vi "RT-Main_withPID.vi"() -> ()   [LabVIEW 2018]
uses:
  <vilib>/Studica/Studica Toolkit/Background/I2C Channel.ctl
  <vilib>/Studica/Studica Toolkit/Background/Mxp Selection.ctl
  <vilib>/robotics/Steering/Wheel/Rotation Direction.ctl
  <vilib>/robotics/Steering/Wheel/Wheel Parameters.ctl
  <vilib>/robotics/Steering/Omnidirectional Wheel/NI_Robotics_Omnidirectional Wheel.lvclass
  C:/Program Files (x86)/National Instruments/LabVIEW 2018/vi.lib/robotics/Steering/Wheel/NI_Robotics_Wheel.lvclass
  <vilib>/robotics/Steering/Omnidirectional Wheel/Create Omnidirectional Wheel.vi
  <vilib>/robotics/Steering/Steering Frame/Create User Defined Steering Frame.vi
  <vilib>/robotics/Steering/Steering Frame/Apply Steering Frame Velocity to Motors.vi
  <vilib>/robotics/Steering/Steering Frame/NI_Robotics_Steering Frame.lvclass
  <vilib>/robotics/Steering/Wheel/NI_Robotics_Wheel.lvclass
  <vilib>/Studica/Studica Toolkit/NavX/NavX.lvlib
  <vilib>/Studica/Studica Blackhawk/Blackhawk.lvlib
panel:
  in  "Robot Facing":i16=4
  out "data out":T1(array[cluster])
  in  "NavX PID gains":T2(array[cluster])=[{"proportional gain (Kc)"=0.15, "integral time (Ti, min)"=0.0, "derivative time (Td, min)"=0.003}] {"integral time (Ti, min)" min=0.0 step=0.0001}
  out "Angular velocity setpoint":dbl
  out "YRPHfH":T3={"Yaw"=0.15, "Roll"=2.38, "Pitch"=-4.28, "Heading"=48.3, "Fused Heading"=0.15}
  out "error out":errorcluster
  in  "Angular Velocity (rad/s)":dbl(slide)=-0.0 min=-1.0 max=1.0 scale=1.0..-1.0
  in  "Y Velocity (m/s)":dbl(slide)=-0.0 min=-1.0 max=1.0 scale=-1.0..1.0
  in  "X Velocity (m/s)":dbl(slide)=-0.0 min=-1.0 max=1.0 scale=-1.0..1.0
  in  "Wheel Index Adjustment":i32[](array[numeric])=[2, 0, 1]
  out "Desired Velocity":dbl[](array[numeric])=[0.0033749999999999995, 0.0033749999999999995, 0.0033749999999999995]
  out "PID-Output":dbl[](array[numeric])=[0.004570312508683128, 0.004570312508683128, 0.004570312508683128, 0.004570312508683128]
  in  "PID gains":T2(array[cluster])=[{"proportional gain (Kc)"=1.3, "integral time (Ti, min)"=0.004, "derivative time (Td, min)"=0.0}, {"proportional gain (Kc)"=1.3, "integral time (Ti, min)"=0.004, "derivative time (Td, min)"=0.0}, {"proportional gain (Kc)"=1.3, "integral time (Ti, min)"=0.004, "derivative time (Td, min)"=0.0}] {"proportional gain (Kc)" step=0.01; "integral time (Ti, min)" min=0.0 step=0.0001; "derivative time (Td, min)" step=0.0001}
  in  "Reset Encoders":bool
  out "Actual-SpeedList":dbl[](array[numeric])
  out "Tick Count(uSec)":u32=10160615 caption="Tick Count(Ticks)"
  in  "Speed M1":dbl(slide) scale=-1.0..1.0
  in  "StopMotors":bool
  in  "Stop Program":bool
  in  "Robot Model":string(combo)="3-wheeled"
  out "timed out?":bool
  out "available IP addresses":string[](array[string])=["172.16.0.1", "127.0.0.1"]
  # "Configuration"
  # "Speed related shit"
  # "Controller"
  # "NAVX data"
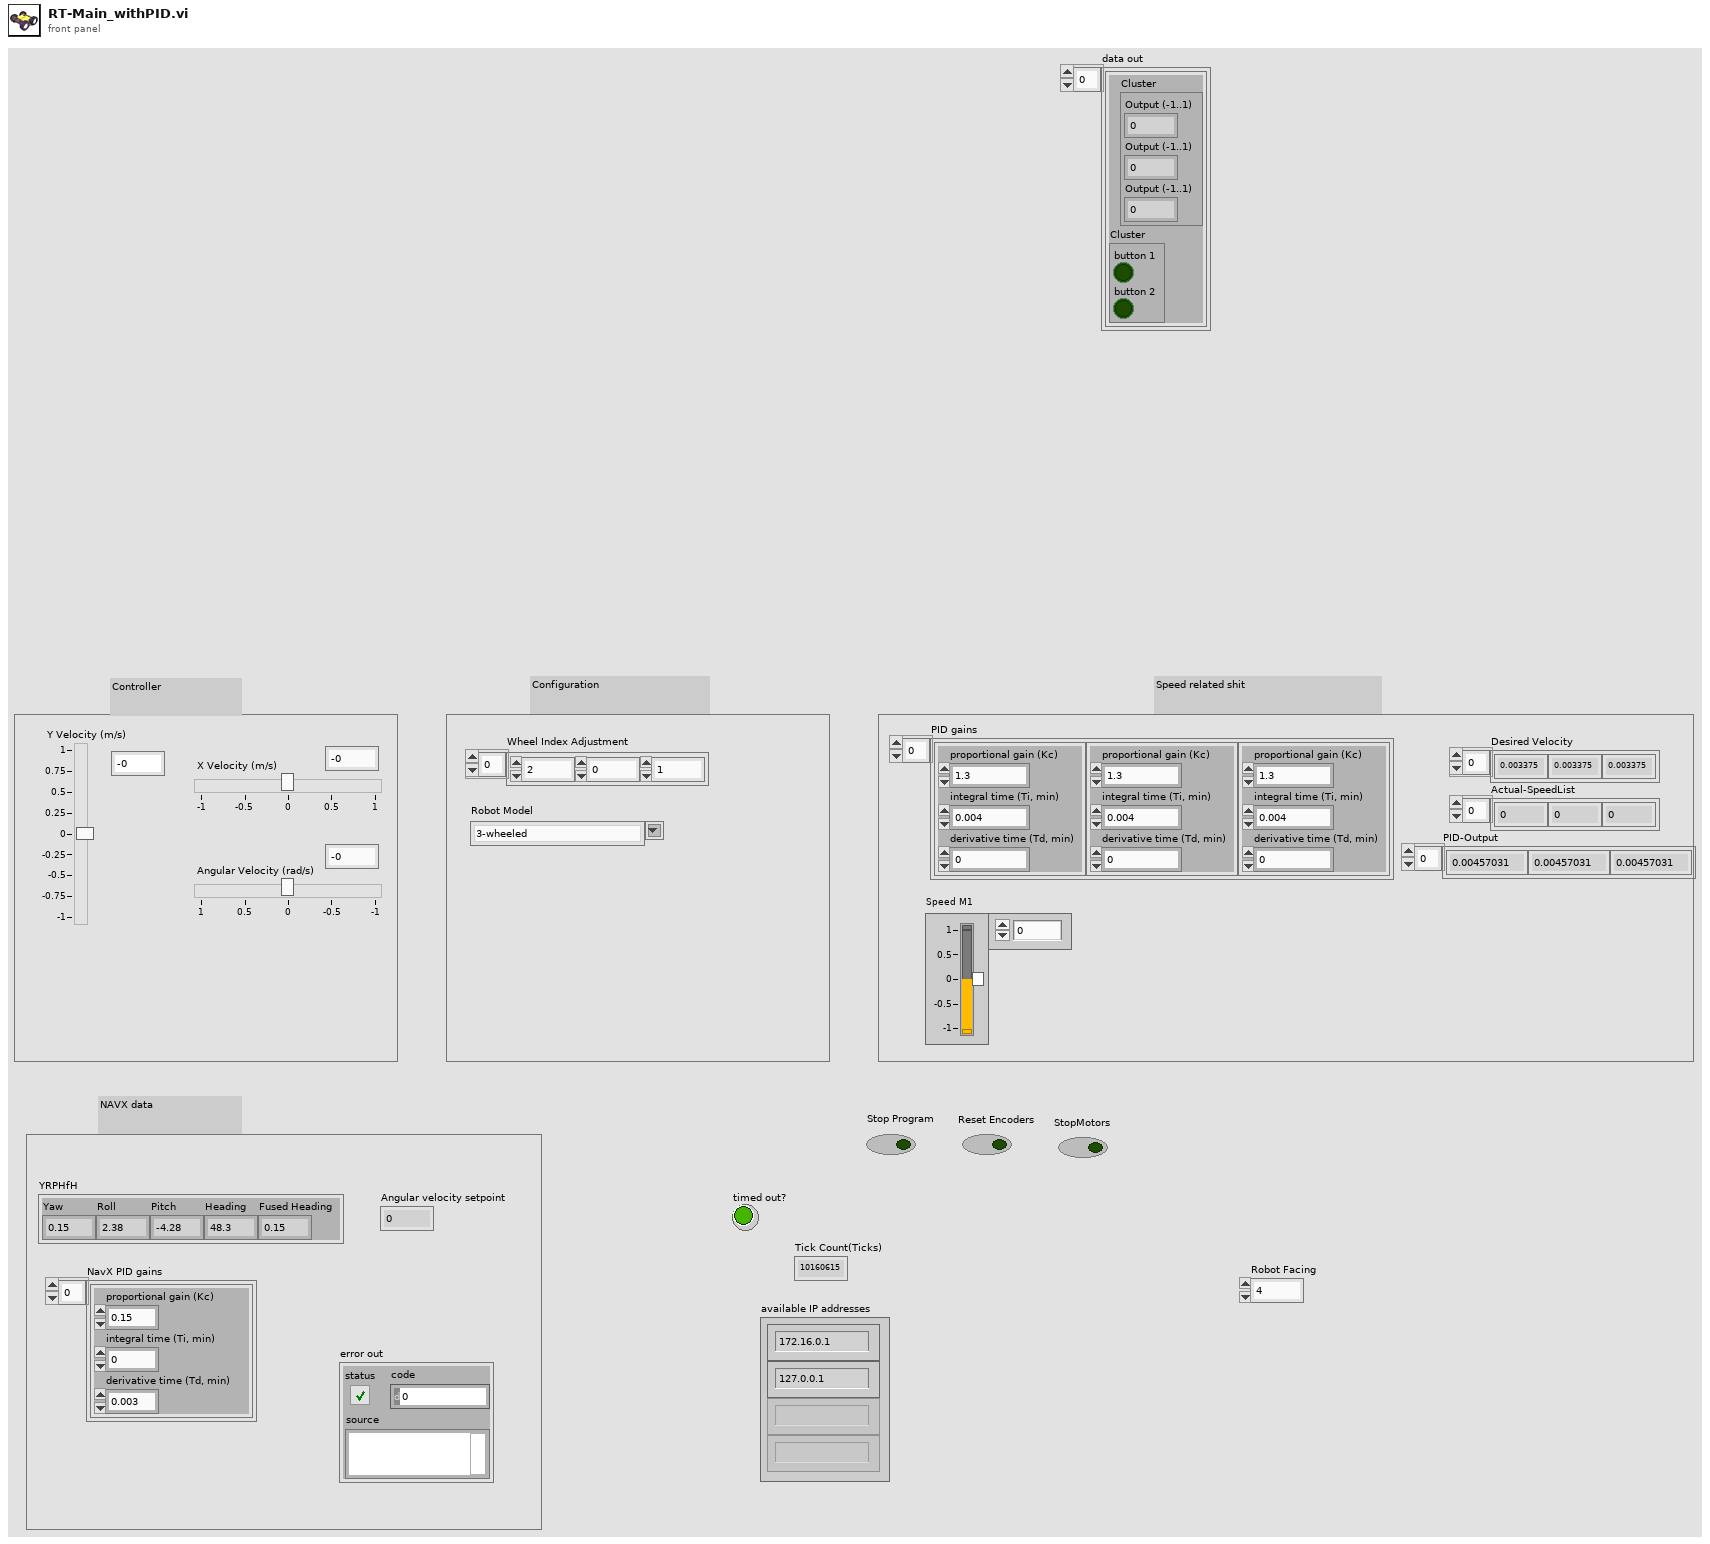
[diagram p1: front panel]
types:
  T1 = cluster{"Cluster":cluster{"Output (-1..1)":dbl, "Output (-1..1)":dbl, "Output (-1..1)":dbl}, "Cluster":cluster{"button 1":bool, "button 2":bool}}[]
  T2 = cluster{"proportional gain (Kc)":dbl, "integral time (Ti, min)":dbl, "derivative time (Td, min)":dbl}[]
  T3 = cluster{"Yaw":dbl, "Roll":dbl, "Pitch":dbl, "Heading":dbl, "Fused Heading":dbl}
  T4 = typedef "I2C Channel.ctl" = enum16{"Not Connected", "A", "B"}
  T5 = cluster{"Cluster":cluster{"Output (-1..1)":dbl, "Output (-1..1)":dbl, "Output (-1..1)":dbl}, "Cluster":cluster{"button 1":bool, "button 2":bool}}
  T6 = cluster{"Output (-1..1)":dbl, "Output (-1..1)":dbl, "Output (-1..1)":dbl}
  T7 = typedef "Mxp Selection.ctl" = enum16{"MXP A", "MXP B"}
  T8 = typedef "I2C.lvlib/I2C Reference.ctl" = cluster{"myRIO Reference":T9, "I2C Channels Enum":T13, "I2C Configuration":T14}
  T9 = typedef "myRIO Generic Hardware Reference.ctl" = cluster{"myRIO Model":T10, "myRIO Hardware Reference":T11}
  T10 = typedef "Hardware Version Enum.ctl" = enum16{"Unknown", "myRIO-1900", "myRIO-1950", "roboRIO", "NI ELVIS RIO CM", "ELVIS III"}
  T11 = typedef "myRIO v1.0 Reference.ctl" = cluster{"Generic FPGA Reference":T12, "Allow multiple opens":bool}
  T12 = typedef "Generic FPGA Reference.ctl" = refnum<k20>
  T13 = typedef "I2C Channels Enum.ctl" = enum16{"Not Connected", "A/I2C", "B/I2C", "I2C/I2C"}
  T14 = typedef "I2C.lvlib/I2C Configuration.ctl" = cluster{"I2C Transfer Rate":T15}
  T15 = typedef "I2C.lvlib/I2C Transfer Rate.ctl" = enum16{"Standard mode (100 kbps)", "Fast mode (400 kbps)"}
  T16 = cluster{"I2C Ref Out":cluster{"I2C Channel":T4, "FPGA VI Reference Out":refnum<k20>}, "Connected":bool, "Slave Address (7-bit)":u8, "Registry":u8[]}
  T17 = typedef "NI_Robotics_Wheel.lvclass/Wheel Parameters.ctl" = cluster{"wheel radius":dbl, "gear ratio":dbl, "forward rotation direction":T18}
  T18 = typedef "NI_Robotics_Wheel.lvclass/Rotation Direction.ctl" = u16
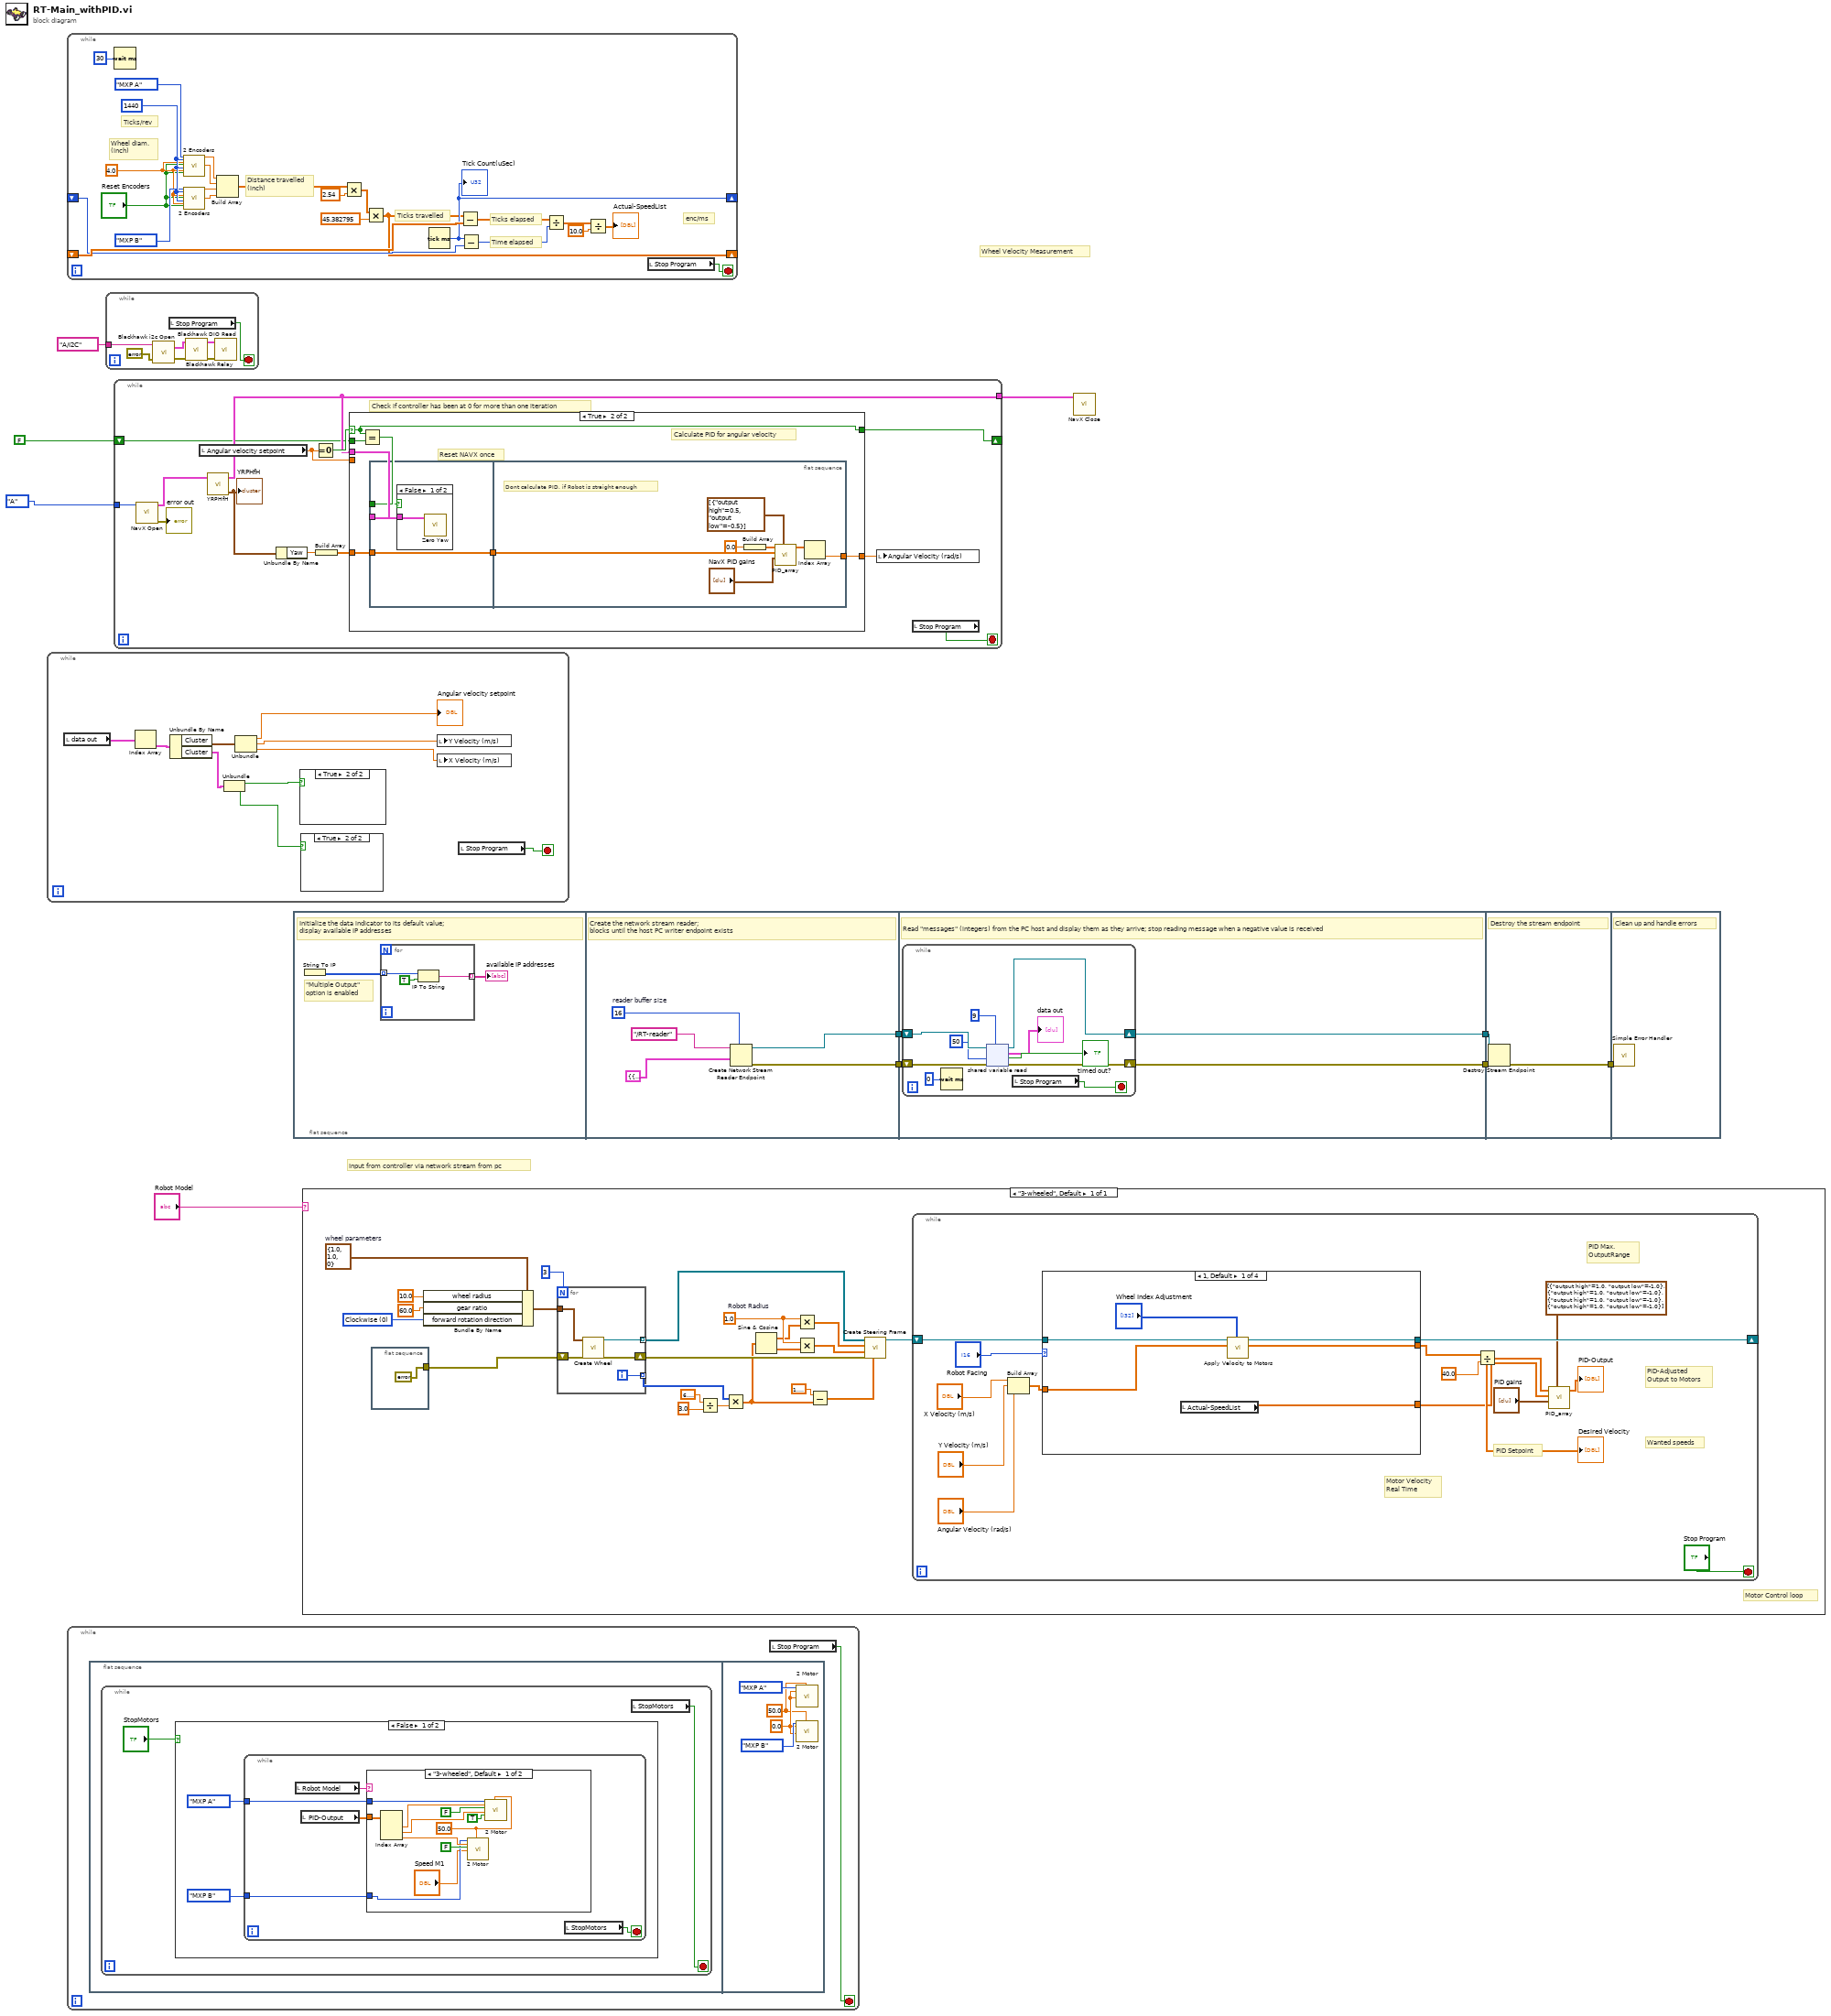
[diagram p0: block diagram]
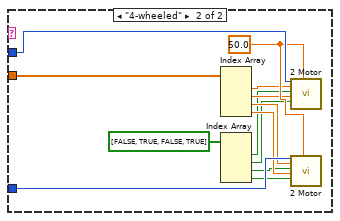
[diagram p6: hidden frame]
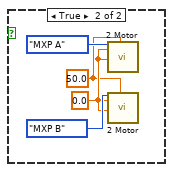
[diagram p7: hidden frame]
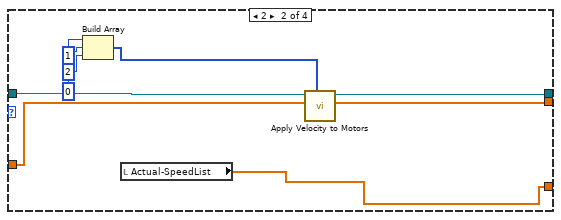
[diagram p8: hidden frame]
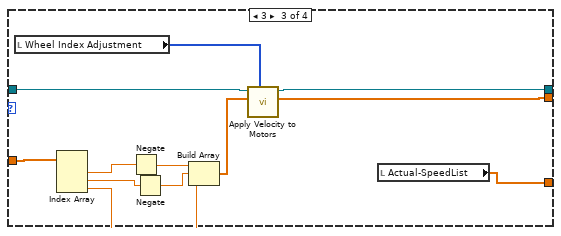
[diagram p9: hidden frame]
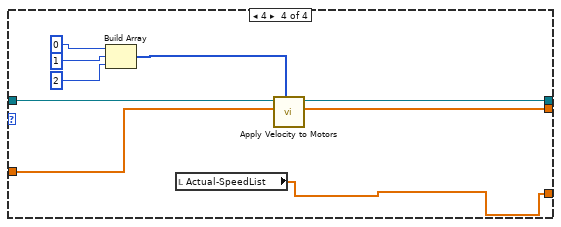
[diagram p10: hidden frame]
diagram:
  # "Input from controller via network stream from pc"
  # "Wheel Velocity Measurement"
  n1 = while {
    stop <- w20 stop-if-true
    n2 = local read "data out"() -> (w19:T1)
    n3 = Index Array(array=w19) -> (element=w18:T5)  [unwired: 1 in]
    n4 = Unbundle By Name(w18) -> ("Cluster"=w17:T6, "Cluster"=w13:cluster{"button 1":bool, "button 2":bool})
    n5 = Unbundle(w13) -> ("button 1"=w12:bool, "button 2"=w11:bool)
    n6 = Unbundle(w17) -> ("Output (-1..1)"=→"Angular velocity setpoint":dbl, "Output (-1..1)"=w15:dbl, "Output (-1..1)"=w14:dbl)
    n7 = case shown="True" w12 {
      frame False {
      }
      frame True {
      }
    }
    n8 = case shown="True" w11 {
      frame False {
      }
      frame True {
      }
    }
    n9 = local write "Y Velocity (m/s)"(w15) -> ()
    n10 = local write "X Velocity (m/s)"(w14) -> ()
    n11 = local read "Stop Program"() -> (w20:bool)
  }
  n12 = while {
    shift-right: [w28] -> _
    shift-left: _ -> [w33]
    shift-right: [w29] -> _
    shift-left: _ -> [w31]
    stop <- w21 stop-if-true
    w26 = 4.0 ("Wheel Diameter M1 (inches)")
    w36 = u32 1440 ("Ticks Per Rev M0")
    # "Ticks travelled"
    # "Distance travelled\n(inch)"
    # "Wheel diam.\n(inch)"
    # "Ticks/rev"
    # "Ticks elapsed"
    # "Time elapsed"
    # "enc/ms"
    n13 = Wait (ms)(milliseconds to wait=u32 30) -> ()  [unwired: 1 out]
    n14 = call <vilib>:"2 Encoders.vi"("Mxp Side"=Mxp_Selection."MXP A", "Ticks Per Rev M0"=w36, "Wheel Diameter M0 (inches)"=w26, "Reset Encoder 0"="Reset Encoders", "Ticks Per Rev M1"=w36, "Wheel Diameter M1 (inches)"=w26, "Reset Encoder 1"="Reset Encoders") -> ("Distance M0 (inches)"=w37:dbl, "Distance M1 (inches)"=w38:dbl)  [unwired: 18 in, 1 out]
    n15 = call <vilib>:"2 Encoders.vi"("Mxp Side"=Mxp_Selection."MXP B", "Ticks Per Rev M0"=w36, "Wheel Diameter M0 (inches)"=w26, "Reset Encoder 0"="Reset Encoders", "Ticks Per Rev M1"=w36, "Wheel Diameter M1 (inches)"=w26, "Reset Encoder 1"="Reset Encoders") -> ("Distance M0 (inches)"=w39:dbl, "Distance M1 (inches)"=w27:dbl)  [unwired: 18 in, 1 out]
    n16 = Build Array(w37, w38, w39, w27) -> (w41:dbl[])
    n17 = Multiply(x=w41, y=2.54) -> (x*y=w42:dbl[])
    n18 = Multiply(x=w42, y=45.382795) -> (x*y=w28:dbl[])
    n19 = Tick Count (ms)() -> (millisecond timer value=w29:u32)
    "Tick Count(uSec)" <- w29
    n20 = Subtract(x=w28, y=w33) -> (x-y=w32:dbl[])
    n21 = Subtract(x=w29, y=w31) -> (x-y=w44:u32)
    n22 = Divide(x=w32, y=w44) -> (x/y=w24:dbl[])
    n23 = Divide(x=w24, y=10.0) -> (x/y=→"Actual-SpeedList":dbl[])
    n24 = local read "Stop Program"() -> (w21:bool)
  }
  n25 = while {
    stop <- w45 stop-if-true
    n26 = flat-sequence {
      frame #0 {
        n27 = while {
          stop <- w46 stop-if-true
          n28 = case shown="False" "StopMotors" {
            frame False {
              n29 = while {
                tunnel: Mxp_Selection."MXP A" ("Mxp Side") -> [w54]
                tunnel: Mxp_Selection."MXP B" ("Mxp Side") -> [w53]
                stop <- w50 stop-if-true
                n30 = local read "Robot Model"() -> (w52:string)
                n31 = local read "PID-Output"() -> (w51:dbl[])
                n32 = case shown="\"3-wheeled\", Default" w52 {
                  tunnel: w54 -> [w57 w78]
                  tunnel: w53 -> [w56 w77]
                  tunnel: w51 -> [w58 w66]
                  frame "3-wheeled", Default {
                    w65 = 50.0 ("Frequency [Hz]")
                    n33 = Index Array(array=w58) -> (element #1=w61:dbl, element #2=w60:dbl, element #3=w59:dbl)  [unwired: 3 in]
                    n34 = call <vilib>:"2 Motor.vi"("Mxp Side"=w56, "Speed M0"=w59, "Invert M0"=FALSE, "Speed M1"="Speed M1", "Frequency [Hz]"=w65) -> ()  [unwired: 14 in, 1 out]
                    n35 = call <vilib>:"2 Motor.vi"("Mxp Side"=w57, "Speed M0"=w61, "Invert M0"=FALSE, "Speed M1"=w60, "Invert M1"=TRUE ("Invert M0"), "Frequency [Hz]"=w65) -> ()  [unwired: 13 in, 1 out]
                  }
                  frame "4-wheeled" {
                    w76 = 50.0 ("Frequency [Hz]")
                    n36 = Index Array(array=w66) -> (element #1=w75:dbl, element #2=w74:dbl, element #3=w73:dbl, element #4=w72:dbl)  [unwired: 4 in]
                    n37 = Index Array(array=bool[] [FALSE, TRUE, FALSE, TRUE] ("Motor Directions")) -> (element #1=w70:bool, element #2=w69:bool, element #3=w68:bool, element #4=w67:bool)  [unwired: 4 in]
                    n38 = call <vilib>:"2 Motor.vi"("Mxp Side"=w78, "Speed M0"=w75, "Invert M0"=w70, "Speed M1"=w74, "Invert M1"=w69, "Frequency [Hz]"=w76) -> ()  [unwired: 13 in, 1 out]
                    n39 = call <vilib>:"2 Motor.vi"("Mxp Side"=w77, "Speed M0"=w73, "Invert M0"=w68, "Speed M1"=w72, "Invert M1"=w67, "Frequency [Hz]"=w76) -> ()  [unwired: 13 in, 1 out]
                  }
                }
                n40 = local read "StopMotors"() -> (w50:bool)
              }
            }
            frame True {
              w79 = 50.0 ("Frequency [Hz]")
              w80 = 0.0 ("Speed M0")
              n41 = call <vilib>:"2 Motor.vi"("Mxp Side"=Mxp_Selection."MXP A", "Speed M0"=w80, "Speed M1"=w80, "Frequency [Hz]"=w79) -> ()  [unwired: 15 in, 1 out]
              n42 = call <vilib>:"2 Motor.vi"("Mxp Side"=Mxp_Selection."MXP B", "Speed M0"=w80, "Speed M1"=w80, "Frequency [Hz]"=w79) -> ()  [unwired: 15 in, 1 out]
            }
          }
          n43 = local read "StopMotors"() -> (w46:bool)
        }
      }
      frame #1 {
        w83 = 50.0 ("Frequency [Hz]")
        w84 = 0.0 ("Speed M0")
        n44 = call <vilib>:"2 Motor.vi"("Mxp Side"=Mxp_Selection."MXP A", "Speed M0"=w84, "Speed M1"=w84, "Frequency [Hz]"=w83) -> ()  [unwired: 15 in, 1 out]
        n45 = call <vilib>:"2 Motor.vi"("Mxp Side"=Mxp_Selection."MXP B", "Speed M0"=w84, "Speed M1"=w84, "Frequency [Hz]"=w83) -> ()  [unwired: 15 in, 1 out]
      }
    }
    n46 = local read "Stop Program"() -> (w45:bool)
  }
  n47 = while {
    tunnel: tag "A/I2C" ("Channel Name") -> [w93]
    stop <- w92 stop-if-true
    n48 = call <vilib>:"Blackhawk i2c Open.vi"("error in (no error)"=errorcluster {"status"=FALSE, "code"=0, "source"=""}, "Channel Name"=w93) -> ("error out"=w89:errorcluster, "I2C Ref Out"=w90:T8)  [unwired: 2 in]
    n49 = local read "Stop Program"() -> (w92:bool)
    n50 = call <vilib>:"Blackhawk Relay.vi"("error in (no error)"=w89, "I2C Ref In"=w90) -> ("error out"=w87:errorcluster, "I2C Ref Out"=w88:T8)  [unwired: 8 in]
    n51 = call <vilib>:"Blackhawk DIO Read.vi"("I2C Ref In"=w88, "error in (no error)"=w87) -> ()  [unwired: 4 in, 3 out]
  }
  n52 = while {
    tunnel: [w98] -> w4
    shift-right: [w96] -> _
    shift-left: FALSE -> [w95]
    tunnel: I2C_Channel."A" ("I2C Channel") -> [w94]
    stop <- w106 stop-if-true
    # "Check if controller has been at 0 for more than one iteration"
    n53 = call <vilib>:"NavX Open.vi"("I2C Channel"=w94) -> ("error out"=→"error out":errorcluster, "NavX Info"=w104:T16)  [unwired: 9 in]
    n54 = local read "Angular velocity setpoint"() -> (w97:dbl)
    n55 = call <vilib>:"YRPHfH.vi"("NavX Info In"=w104) -> ("YRPHfH"=w103:T3, "NavX Info Out"=w98:T16)  [unwired: 3 in]
    "YRPHfH" <- w103
    n56 = Unbundle By Name(w103) -> ("Yaw"=w99:dbl)
    n57 = Equal To 0?(x=w97) -> (x = 0?=w100:bool)
    n58 = Build Array(w99) -> (w102:dbl[])
    n59 = case shown="True" w100 {
      selector: w100 -> [w107 w111]
      tunnel: w102 -> [_ w114]
      tunnel: [w108 w115] -> w101
      tunnel: w98 -> [_ w112]
      tunnel: w97 -> [w108 _]
      tunnel: [w107 w111] -> w96
      tunnel: w95 -> [_ w110]
      frame False {
        # "Adjust angular velocity if controller != 0"
      }
      frame True {
        # "Reset NAVX once"
        # "Calculate PID for angular velocity"
        n60 = Equal?(x=w111, y=w110) -> (x = y?=w109:bool)
        n61 = flat-sequence {
          tunnel: [w118] -> w113
          tunnel: w114 -> [w118]
          tunnel: w112 -> [w117]
          tunnel: w109 -> [w116]
          tunnel: [w126] -> w115
          tunnel: w113 -> [w125]
          frame #0 {
            n62 = case shown="False" w116 {
              tunnel: w117 -> [w119 _]
              frame False {
                n63 = call <vilib>:"Zero Yaw.vi"("NavX Info In"=w119) -> ()  [unwired: 10 in, 1 out]
              }
              frame True {
              }
            }
          }
          frame #1 {
            # "Dont calculate PID, if Robot is straight enough"
            n64 = Build Array(0.0 ("element")) -> (w123:dbl[])
            n65 = call "PID_array.vi"("output range"=cluster{"output high":dbl, "output low":dbl}[] [{"output high"=0.5, "output low"=-0.5}], "PID gains"="NavX PID gains", "process variable"=w125, "setpoint"=w123) -> ("output"=w124:dbl[])  [unwired: 6 in, 1 out]
            n66 = Index Array(array=w124) -> (element=w126:dbl)  [unwired: 1 in]
          }
        }
      }
    }
    n67 = local write "Angular Velocity (rad/s)"(w101) -> ()
    n68 = local read "Stop Program"() -> (w106:bool)
  }
  n69 = flat-sequence {
    tunnel: [w134] -> w10
    tunnel: [w133] -> w9
    tunnel: [w137] -> w8
    tunnel: [w138] -> w7
    tunnel: w10 -> [w139]
    tunnel: w9 -> [w140]
    tunnel: w8 -> [w153]
    tunnel: w7 -> [w152]
    tunnel: [w151] -> w6
    tunnel: w6 -> [w154]
    frame #0 {
      # "\"Multiple Output\"\noption is enabled"
      # "Initialize the data indicator to its default value;\ndisplay available IP addresses"
      n70 = String To IP() -> (0:w127:u32[])  [unwired: 1 in]
      n71 = for {
        tunnel: w127 -> [w130] mode=indexing
        tunnel: [w129] -> w128 mode=indexing
        n72 = IP To String(1:TRUE ("dot notation? (F)"), 2:w130) -> (0:w129:string)
      }
      "available IP addresses" <- w128
    }
    frame #1 {
      w136 = 16  # reader buffer size
      # "Create the network stream reader;\nblocks until the host PC writer endpoint exists"
      n73 = Create Network Stream Reader Endpoint(7:w136, 9:T5 {"Cluster"={"Output (-1..1)"=0.0, "Output (-1..1)"=0.0, "Output (-1..1)"=0.0}, "Cluster"={"button 1"=FALSE, "button 2"=FALSE}} ("Controller Values"), 11:"/RT-reader" ("writer name")) -> (0:w134:errorcluster, 3:w133:refnum<k21>)  [unwired: 4 in]
    }
    frame #2 {
      # "Read \"messages\" (integers) from the PC host and display them as they arrive; stop reading message when a negative value is received"
      n74 = while {
        shift-right: [w148] -> w137
        shift-left: w140 -> [w150]
        shift-right: [w144] -> w138
        shift-left: w139 -> [w147]
        stop <- w142 stop-if-true
        n75 = Wait (ms)(milliseconds to wait=u32 0) -> ()  [unwired: 1 out]
        n76 = shared-variable-read(w150, w147, 50 ("timeout ms (-1)"), 9 ("# elements")) -> (w148:refnum<k21>, w144:errorcluster, →"timed out?":bool, →"data out":T1)
        n77 = local read "Stop Program"() -> (w142:bool)
      }
    }
    frame #3 {
      # "Destroy the stream endpoint"
      n78 = Destroy Stream Endpoint(8:w152, 11:w153) -> (0:w151:errorcluster)
    }
    frame #4 {
      # "Clean up and handle errors"
      n79 = call <vilib>:"Simple Error Handler.vi"("error in (no error)"=w154) -> ()  [unwired: 4 in, 5 out]
    }
  }
  n80 = case shown="\"3-wheeled\", Default" "Robot Model" {
    frame "3-wheeled", Default {
      w176 = T17 {"wheel radius"=1.0, "gear ratio"=1.0, "forward rotation direction"=0}  # wheel parameters
      w161 = T18 0 items=["Clockwise", "Counterclockwise"] ("forward rotation direction")
      w166 = 1.0  # Robot Radius
      # "Motor Control loop"
      n81 = flat-sequence {
        tunnel: [errorcluster {"status"=FALSE, "code"=0, "source"=""} ("error out")] -> w172
        frame #0 {
        }
      }
      n82 = Bundle By Name(cluster=w176, "wheel radius"=10.0, "gear ratio"=60.0, "forward rotation direction"=w161) -> (w173:T17)
      n83 = for {
        N: 3 -> [_]
        shift-right: [w232] -> w159
        shift-left: w172 -> [w233]
        tunnel: [w231] -> w171 mode=indexing
        tunnel: w173 -> [w230]
        tunnel: [w229] -> w167 mode=indexing
        i -> [w229]
        n84 = call-poly <vilib>:"Create Wheel.vi"("error in (no error)"=w233, "wheel parameters"=w230) -> ("error out"=w232:errorcluster, "omni wheel out"=w231:refnum<class "NI_Robotics_Omnidirectional Wheel.lvclass">)  [unwired: 8 in]
      }
      n85 = Divide(x=6.283185307179586, y=3.0) -> (x/y=w168:dbl)
      n86 = Multiply(x=w167, y=w168) -> (x*y=w156:dbl[])
      n87 = Sine & Cosine(0:w156) -> (1:w158:dbl[], 2:w157:dbl[])
      n88 = Multiply(x=w166, y=w158) -> (x*y=w165:dbl[])
      n89 = Multiply(x=w166, y=w157) -> (x*y=w164:dbl[])
      n90 = Subtract(x=1.5707963267948966, y=w156) -> (x-y=w162:dbl[])
      n91 = call-poly <vilib>:"Create Steering Frame.vi"("wheel frame angles (rad)"=w162, "error in (no error)"=w159, "wheel y positions"=w164, "wheel x positions"=w165, "wheels"=w171) -> ("steering frame out"=w155:refnum<class "NI_Robotics_Steering Frame.lvclass">)  [unwired: 5 in, 1 out]
      n92 = while {
        shift-right: [w191] -> _
        shift-left: w155 -> [w178]
        stop <- "Stop Program" stop-if-true
        # "Wanted speeds"
        # "PID-Adjusted\nOutput to Motors"
        # "Motor Velocity\nReal Time"
        # "PID Max. \nOutputRange"
        # "PID Setpoint"
        n93 = Build Array("X Velocity (m/s)", "Y Velocity (m/s)", "Angular Velocity (rad/s)") -> (w179:dbl[])
        n94 = case shown="1, Default" "Robot Facing" {
          tunnel: w178 -> [w197 w206 w217 w226]
          tunnel: [w196 w205 w218 w225] -> w191
          tunnel: [w194 w203 w215 w224] -> w190
          tunnel: [w193 w198 w207 w219] -> w187
          tunnel: w179 -> [w192 w204 w214 w227]
          frame 1, Default {
            n95 = local read "Actual-SpeedList"() -> (w193:dbl[])
            n96 = call-poly <vilib>:"Apply Velocity to Motors.vi"("wheel indexes"="Wheel Index Adjustment", "steering frame velocity"=w192, "steering frame in"=w197) -> ("ccw motor velocity setpoints"=w194:dbl[], "steering frame out"=w196:refnum<class "NI_Robotics_Steering Frame.lvclass">)  [unwired: 4 in, 3 out]
          }
          frame 2 {
            n97 = Build Array(1, 2, 0) -> (w199:i32[])
            n98 = local read "Actual-SpeedList"() -> (w198:dbl[])
            n99 = call-poly <vilib>:"Apply Velocity to Motors.vi"("wheel indexes"=w199, "steering frame velocity"=w204, "steering frame in"=w206) -> ("ccw motor velocity setpoints"=w203:dbl[], "steering frame out"=w205:refnum<class "NI_Robotics_Steering Frame.lvclass">)  [unwired: 4 in, 3 out]
          }
          frame 3 {
            n100 = local read "Wheel Index Adjustment"() -> (w216:i32[])
            n101 = Index Array(array=w214) -> (element #1=w213:dbl, element #2=w212:dbl, element #3=w209:dbl)  [unwired: 3 in]
            n102 = Negate(x=w213) -> (-x=w211:dbl)
            n103 = Negate(x=w212) -> (-x=w210:dbl)
            n104 = Build Array(w211, w210, w209) -> (w208:dbl[])
            n105 = call-poly <vilib>:"Apply Velocity to Motors.vi"("wheel indexes"=w216, "steering frame velocity"=w208, "steering frame in"=w217) -> ("ccw motor velocity setpoints"=w215:dbl[], "steering frame out"=w218:refnum<class "NI_Robotics_Steering Frame.lvclass">)  [unwired: 4 in, 3 out]
            n106 = local read "Actual-SpeedList"() -> (w207:dbl[])
          }
          frame 4 {
            n107 = Build Array(0, 1, 2) -> (w220:i32[])
            n108 = local read "Actual-SpeedList"() -> (w219:dbl[])
            n109 = call-poly <vilib>:"Apply Velocity to Motors.vi"("wheel indexes"=w220, "steering frame velocity"=w227, "steering frame in"=w226) -> ("ccw motor velocity setpoints"=w224:dbl[], "steering frame out"=w225:refnum<class "NI_Robotics_Steering Frame.lvclass">)  [unwired: 4 in, 3 out]
          }
        }
        n110 = Divide(x=w190, y=40.0 ("Wheel Diameter M1 (inches)")) -> (x/y=w188:dbl[])
        "Desired Velocity" <- w188
        n111 = call "PID_array.vi"("output range"=cluster{"output high":dbl, "output low":dbl}[] [{"output high"=1.0, "output low"=-1.0}, {"output high"=1.0, "output low"=-1.0}, {"output high"=1.0, "output low"=-1.0}, {"output high"=1.0, "output low"=-1.0}], "PID gains"="PID gains", "process variable"=w187, "setpoint"=w188) -> ("output"=→"PID-Output":dbl[])  [unwired: 6 in, 1 out]
      }
    }
  }
  n112 = call <vilib>:"NavX Close.vi"("NavX Info In"=w4) -> ()  [unwired: 10 in, 1 out]
